vi "Compute_Hierarchy_For_App.vi"(8 "error in (no error)":errorcluster, 10 "sourcePath":path, 11 "AB_Destination in":refnum<class "AB_Destination.lvclass">) -> (0 "error out":errorcluster, 1 "relative to AppDir":bool, 2 "destinationPath":path, 3 "AB_Destination out":refnum<class "AB_Destination.lvclass">)   [LabVIEW 2020, in "AB_Destination.lvclass"]
uses:
  <vilib>/AppBuilder/AB_Classes/Destination/AB_Destination.lvclass
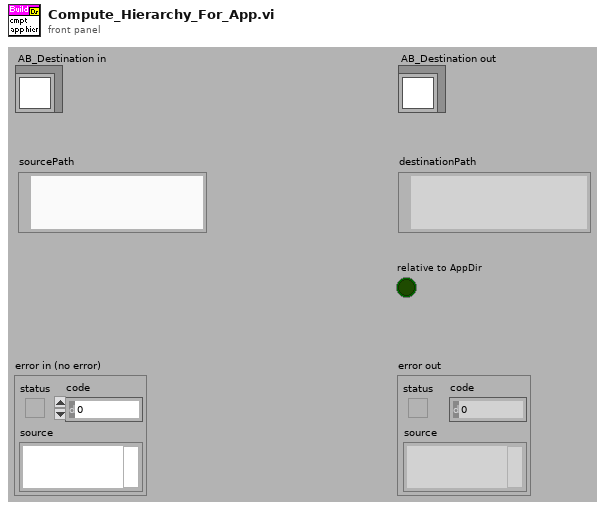
[diagram p1: front panel]
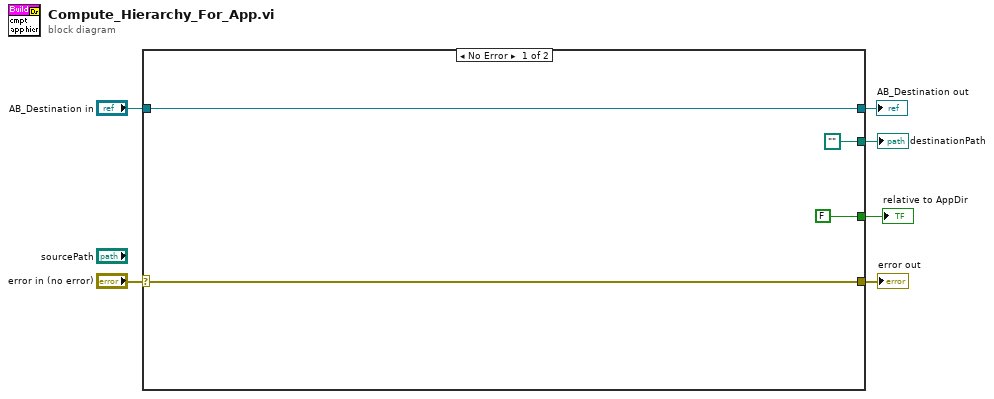
[diagram p0: block diagram]
diagram:
  n1 = case shown="No Error" "error in (no error)" {
    selector: "error in (no error)" -> [w9 w12]
    tunnel: [w9 w12] -> w5
    tunnel: [w10 w11] -> w3
    tunnel: "AB_Destination in" -> [w10 w11]
    tunnel: [path "" _] -> w2
    tunnel: [FALSE _] -> w1
    frame No Error {
    }
    frame Error {
    }
  }
  "error out" <- w5
  "AB_Destination out" <- w3
  "destinationPath" <- w2
  "relative to AppDir" <- w1
